vi "FPGA_laser_control_Qudi.vi"() -> ()   [LabVIEW 2015]
uses:
  <vilib>/rvi/eio/common/nirviEmuTemplateMethod_errors.vi
  <vilib>/eio/EIONode/EIONode.xnode
panel:
  out "value":i16
  in  "561":i16
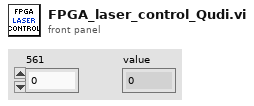
[diagram p1: front panel]
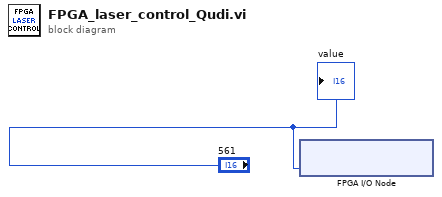
[diagram p0: block diagram]
diagram:
  n1 = xnode "FPGA I/O Node"("Connector0/AO0"="561") -> ()  [unwired: 1 in, 1 out]
  "value" <- "561"
